vi "BandFilter.vi"(10 "IIR filter specifications":T1={"Topology"=enum."Butterworth", "Type"=enum."Bandpass", "Order"=10, "Lower Fc"=3.5, "Upper Fc"=7.5, "PB Ripple"=1.0, "SB Attenuation"=60.0}, 11 "Right Lobe EEG":dynamicdata(waveform)) -> (1 "PSD":cluster{"f0":dbl, "df":dbl, "magnitude":dbl[]}[](array[cluster]), 2 "signal(s) out":waveform(dbl)[](array[waveform]), 3 "mean":dbl)   [LabVIEW 2019]
uses:
  <vilib>/Analysis/baseanly.llb/Mean (DBL).vi
  <vilib>/measure/macond.llb/IIR Filter for N Chan.vi
  <vilib>/express/express analysis/Spectral/Block/exnSpectralBlock spectral measurements PSD poly.vi
  <vilib>/express/express analysis/Spectral/Block/exnSpectralBlock spectral measurements PSD array WFM.vi
  <vilib>/express/express analysis/Spectral/XNode/ExpressSpectralMeasurementsBlockNode.xnode
  <vilib>/measure/NI_MAPro.lvlib
  <vilib>/Analysis/NI_AALBase.lvlib
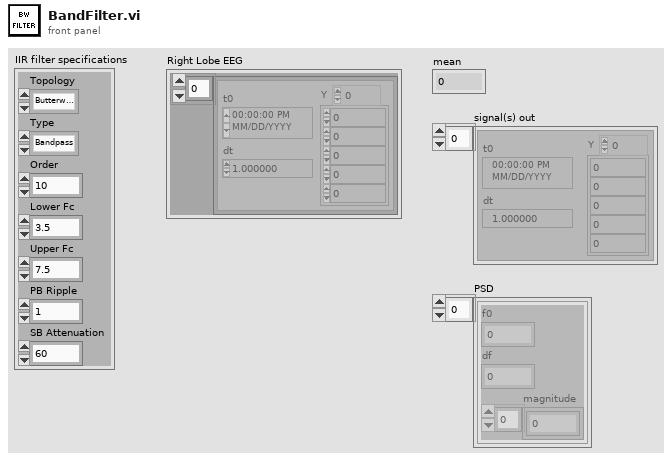
[diagram p1: front panel]
types:
  T1 = cluster{"Topology":enum16{"Off", "Butterworth", "Chebyshev", "Inverse Chebyshev", "Elliptic", "Bessel"}, "Type":enum16{"Lowpass", "Highpass", "Bandpass", "Bandstop"}, "Order":i32, "Lower Fc":dbl, "Upper Fc":dbl, "PB Ripple":dbl, "SB Attenuation":dbl}
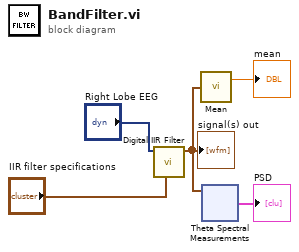
[diagram p0: block diagram]
diagram:
  n1 = call-poly <vilib>:"Digital IIR Filter.vi"("IIR filter specifications"="IIR filter specifications", "signal(s) in"="Right Lobe EEG") -> ("signal(s) out"=w3:waveform(dbl)[])  [unwired: 7 in, 2 out]
  "signal(s) out" <- w3
  n2 = call-poly <vilib>:"Mean.vi"("X"=w3) -> ("mean"=→"mean":dbl)  [unwired: 1 out]
  n3 = xnode ("Theta Spectral Measurements")("Signals"=w3) -> ("PSD"=→"PSD":cluster{"f0":dbl, "df":dbl, "magnitude":dbl[]}[])  [unwired: 1 in, 1 out]
